vi "IFA300Command.vi"(4 "Channel Name":string, 6 "Port Name":string, 8 "ValueToSet":string, 9 "IFACommand":T2="Version", 10 "Address":i8=-1) -> (0 "String Reply":string, 1 "Error Description":string, 2 "Numeric Reply":dbl)   [LabVIEW 2021]
uses:
  IFA300CommandDescriptor.ctl
  IFA300Command.ctl
  IFA300CommandPhases.ctl
panel:
  out "CommandDescriptorOutput":T1
  out "Audit trail":string[](array[string])
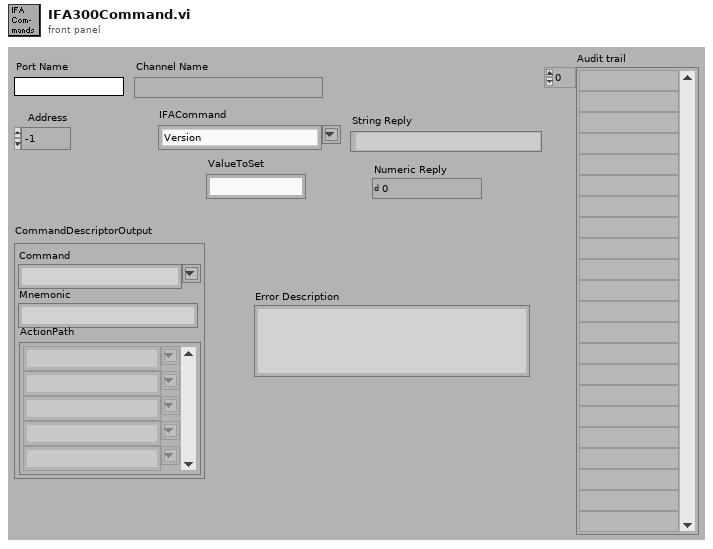
[diagram p1: front panel]
types:
  T1 = typedef "IFA300CommandDescriptor.ctl" = cluster{"Command":T2, "Mnemonic":string, "ActionPath":T3[]}
  T2 = typedef "IFA300Command.ctl" = string
  T3 = typedef "IFA300CommandPhases.ctl" = string
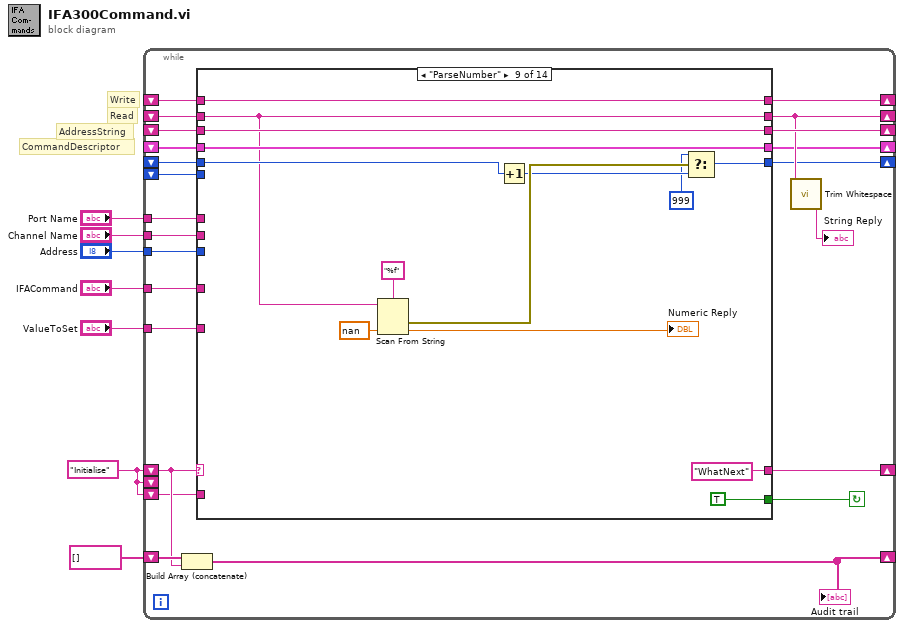
[diagram p0: block diagram]
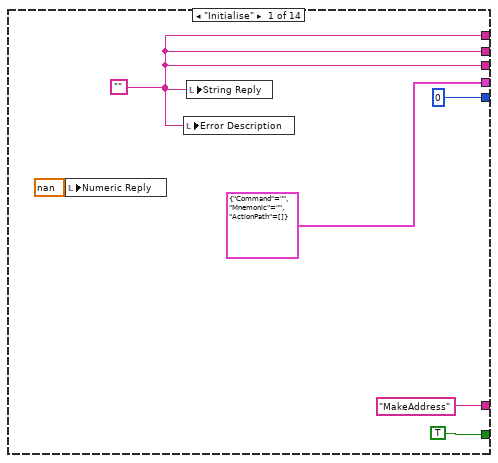
[diagram p2: hidden frame]
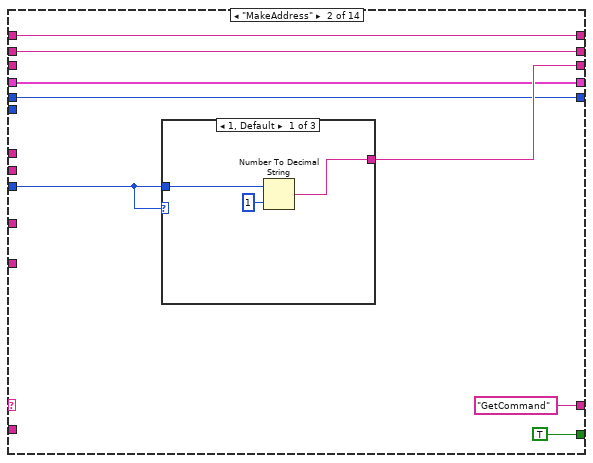
[diagram p3: hidden frame]
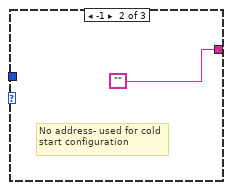
[diagram p4: hidden frame]
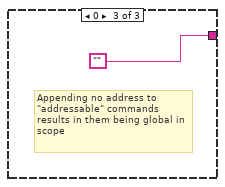
[diagram p5: hidden frame]
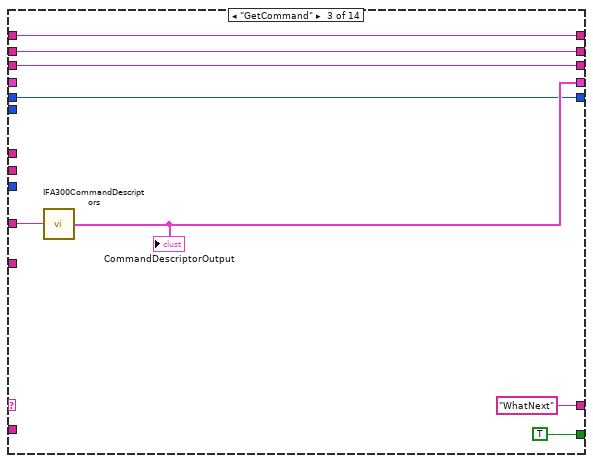
[diagram p6: hidden frame]
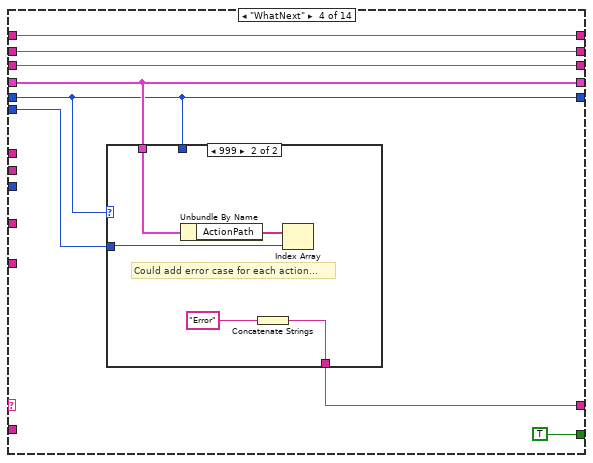
[diagram p7: hidden frame]
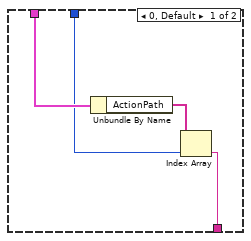
[diagram p8: hidden frame]
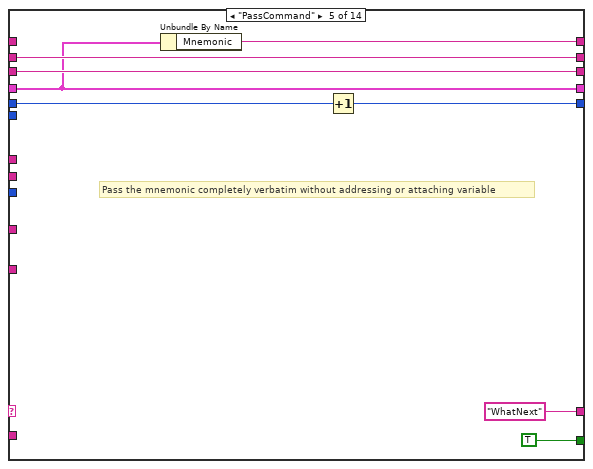
[diagram p9: hidden frame]
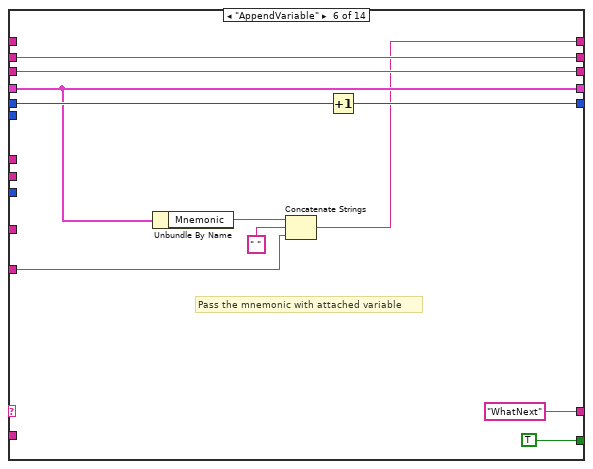
[diagram p10: hidden frame]
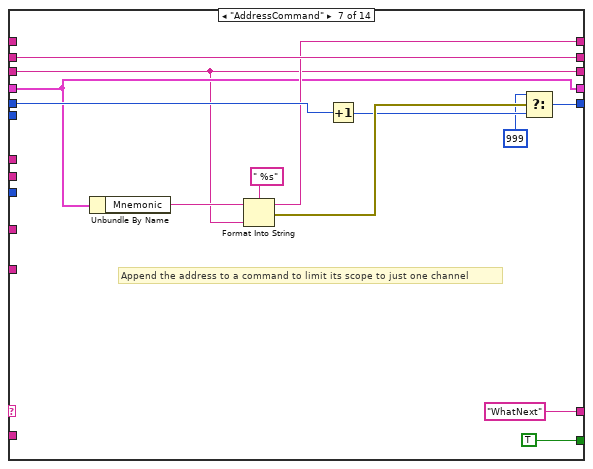
[diagram p11: hidden frame]
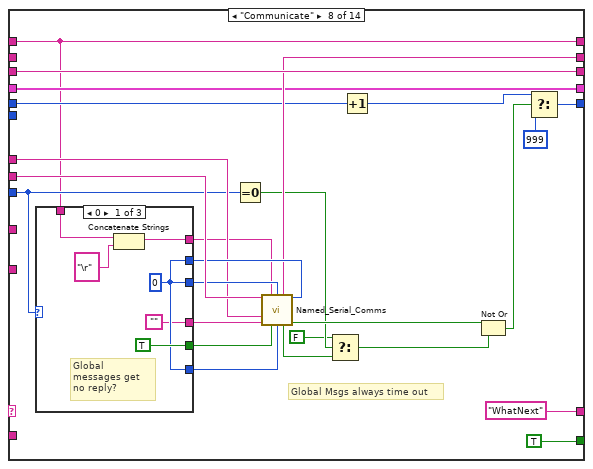
[diagram p12: hidden frame]
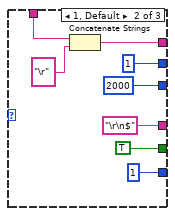
[diagram p13: hidden frame]
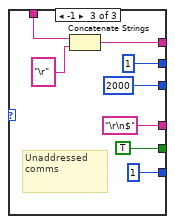
[diagram p14: hidden frame]
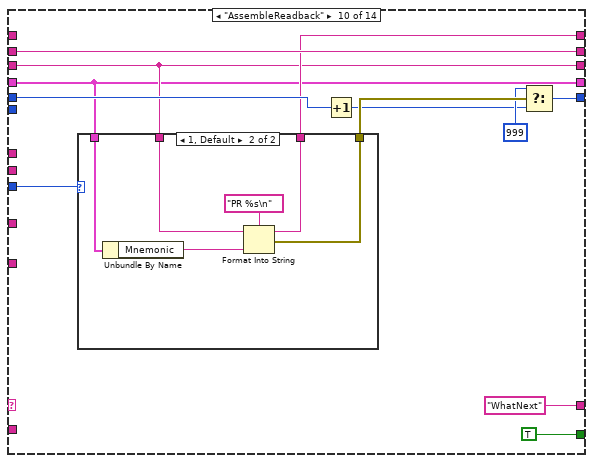
[diagram p15: hidden frame]
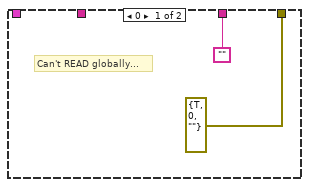
[diagram p16: hidden frame]
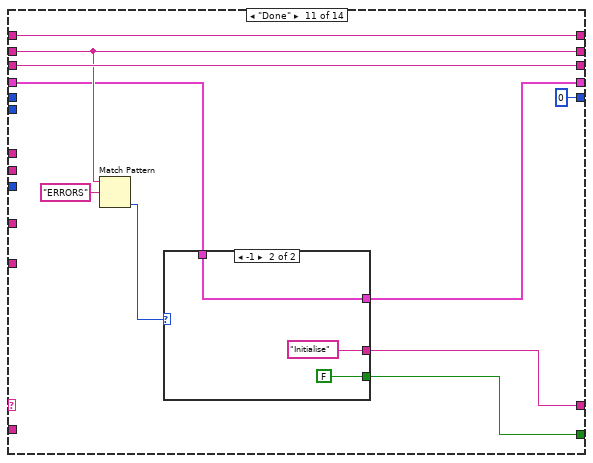
[diagram p17: hidden frame]
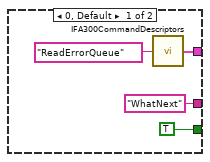
[diagram p18: hidden frame]
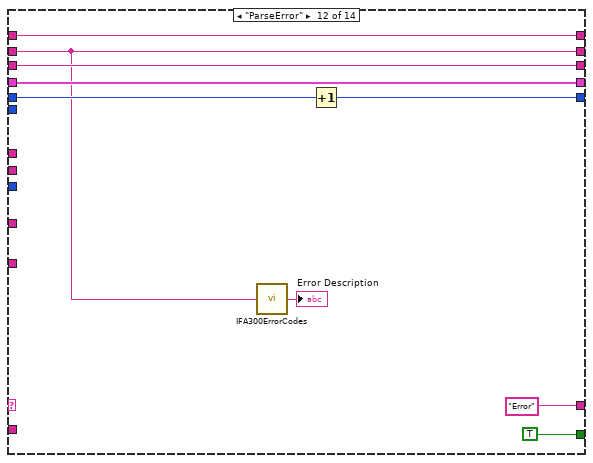
[diagram p19: hidden frame]
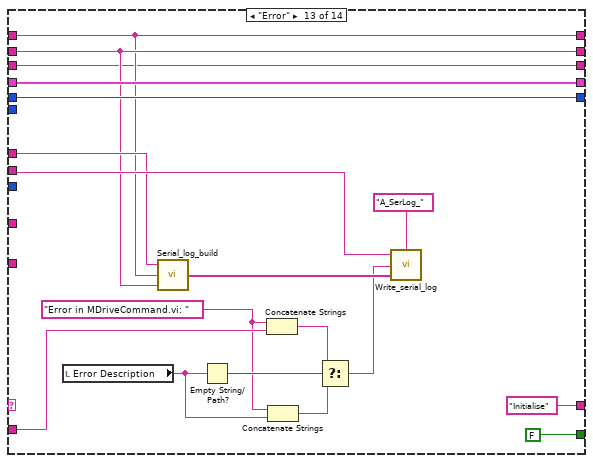
[diagram p20: hidden frame]
diagram:
  w1 = "Initialise"
  # "CommandDescriptor"
  # "AddressString"
  # "Read"
  # "Write"
  n1 = while {
    shift-right: [w18] -> _
    shift-left: w1 -> [w11]
    tunnel: "Address" -> [w30]
    tunnel: "IFACommand" -> [w29]
    tunnel: "ValueToSet" -> [w28]
    shift-right: [w27] -> _
    shift-left: _ -> [w26]
    tunnel: "Port Name" -> [w25]
    tunnel: "Channel Name" -> [w24]
    shift-right: [w16] -> _
    shift-left: _ -> [w23]
    shift-right: [w21] -> _
    shift-left: _ -> [w20]
    shift-right: [w17] -> _
    shift-left: string[] [] -> [w19]
    shift-right: [w15] -> _
    shift-left: _ -> [w14]
    shift-right: [w12] -> _
    shift-left: _ -> [w13]
    shift-left: _ -> [w10]
    shift-left: w1 -> [_]
    shift-left: w1 -> [w9]
    stop <- w22 continue-if-true
    n2 = Build Array (concatenate)(w19, w11) -> (w17:T3[])
    "Audit trail" <- w17
    n3 = case shown="\"ParseNumber\"" w11 {
      selector: w11 -> [_ _ _ _ _ _ _ _ _ _ _ _ _ w236]
      tunnel: ["MakeAddress" "GetCommand" "WhatNext" w61 "WhatNext" "WhatNext" "WhatNext" "WhatNext" "WhatNext" "WhatNext" w191 "Error" "Initialise" w236] -> w18
      tunnel: w30 -> [_ w37 _ _ _ _ _ w109 _ w171 _ _ _ _]
      tunnel: w29 -> [_ _ w54 _ _ _ _ _ _ _ _ _ _ _]
      tunnel: w28 -> [_ _ _ _ _ w83 _ _ _ _ _ _ _ _]
      tunnel: [w31 w42 w56 w64 w76 w85 w101 w108 w155 w174 w197 w208 w215 w234] -> w27
      tunnel: w26 -> [_ w42 w56 w64 _ _ _ w108 w155 _ w197 w208 w215 _]
      tunnel: w25 -> [_ _ _ _ _ _ _ w125 _ _ _ _ w224 _]
      tunnel: w24 -> [_ _ _ _ _ _ _ w131 _ _ _ _ w225 _]
      tunnel: [w31 w41 w55 w63 w82 w93 w106 w122 w161 w179 w195 w205 w216 w234] -> w16
      tunnel: w23 -> [_ w41 w55 w63 w82 w93 w106 _ w161 w179 w195 w205 w216 _]
      tunnel: [TRUE TRUE ("Continue") TRUE ("Continue") TRUE ("Continue") TRUE TRUE TRUE TRUE TRUE TRUE w192 TRUE FALSE ("Continue") FALSE] -> w22
      tunnel: [w31 w44 w53 w62 w78 w89 w94 w123 w166 w172 w196 w212 w214 w234] -> w21
      tunnel: w20 -> [_ _ w53 w62 w78 w89 w94 w123 w166 w172 w196 w212 w214 _]
      tunnel: [T1 {"Command"="", "Mnemonic"="", "ActionPath"=[]} ("CommandDescriptorOutput") w39 w51 w60 w77 w88 w99 w121 w162 w170 w189 w209 w229 w233] -> w15
      tunnel: w14 -> [_ w39 _ w60 w77 w88 w99 w121 w162 w170 w188 w209 w229 w233]
      tunnel: w13 -> [_ w38 w50 w59 w79 w90 w102 w116 w163 w175 _ w210 w228 w232]
      tunnel: [0 w38 w50 w59 w75 w87 w103 w118 w164 w176 0 ("f") w206 w228 w232] -> w12
      tunnel: w10 -> [_ _ _ w58 _ _ _ _ _ _ _ _ _ _]
      tunnel: w9 -> [_ _ _ _ _ _ _ _ _ _ _ _ w222 _]
      frame "Initialise" {
        w31 = ""
        n4 = local write "Numeric Reply"(nan ("Numeric Reply")) -> ()
        n5 = local write "Error Description"(w31) -> ()
        n6 = local write "String Reply"(w31) -> ()
      }
      frame "MakeAddress" {
        n7 = case shown="1, Default" w37 {
          tunnel: w37 -> [w46 _ _]
          tunnel: [w45 "" ""] -> w44
          frame 1, Default {
            n8 = Number To Decimal String(number=w46, width (-)=i16 1) -> (decimal integer string=w45:string)
          }
          frame -1 {
            # "No address- used for cold start configuration"
          }
          frame 0 {
            # "Appending no address to \"addressable\" commands results in them being global in scope"
          }
        }
      }
      frame "GetCommand" {
        n9 = call "IFA300CommandDescriptors.vi"("IFACommand"=w54) -> ("CommandDescriptorOutput"=w51:T1)  [unwired: 4 out]
        "CommandDescriptorOutput" <- w51
      }
      frame "WhatNext" {
        n10 = case shown="999" w59 {
          tunnel: [w68 w71] -> w61
          tunnel: w60 -> [w67 w72]
          tunnel: w59 -> [w66 _]
          tunnel: w58 -> [_ w73]
          frame 0, Default {
            n11 = Unbundle By Name(w67) -> ("ActionPath"=w69:T3[])
            n12 = Index Array(array=w69, index=w66) -> (element=w68:T3)
          }
          frame 999 {
            # "Could add error case for each action..."
            n13 = Unbundle By Name(w72) -> ("ActionPath"=w74:T3[])
            n14 = Concatenate Strings("Error") -> (w71:string)
            n15 = Index Array(array=w74, index=w73) -> ()  [unwired: 1 out]
          }
        }
      }
      frame "PassCommand" {
        # "Pass the mnemonic completely verbatim without addressing or attaching variable"
        n16 = Unbundle By Name(w77) -> ("Mnemonic"=w76:string)
        n17 = Increment(x=w79) -> (x+1=w75:i32)
      }
      frame "AppendVariable" {
        # "Pass the mnemonic with attached variable"
        n18 = Unbundle By Name(w88) -> ("Mnemonic"=w86:string)
        n19 = Concatenate Strings(w86, " " ("string"), w83) -> (w85:string)
        n20 = Increment(x=w90) -> (x+1=w87:i32)
      }
      frame "AddressCommand" {
        # "Append the address to a command to limit its scope to just one channel"
        n21 = Unbundle By Name(w99) -> ("Mnemonic"=w95:string)
        n22 = Format Into String(format string=" %s", initial string=w95, w94) -> (resulting string=w101:string, error out=w98:errorcluster)  [unwired: 1 in]
        n23 = Increment(x=w102) -> (x+1=w97:i32)
        n24 = Select(t=999 ("f"), s=w98, f=w97) -> (s? t:f=w103:i32)
      }
      frame "Communicate" {
        # "Global Msgs always time out"
        n25 = case shown="0" w109 {
          tunnel: ["" "\r\n$" "\r\n$"] -> w130
          tunnel: [w136 1 ("Terminate Count") 1 ("Terminate Count")] -> w129
          tunnel: [w136 u32 2000 ("Timeout/ms") u32 2000 ("Timeout/ms")] -> w128
          tunnel: [TRUE ("Log Errors?") TRUE ("Log Errors?") TRUE ("Log Errors?")] -> w127
          tunnel: [w136 1 ("!Error retries") 1 ("!Error retries")] -> w126
          tunnel: w108 -> [w132 w140 w148]
          tunnel: [w133 w139 w147] -> w107
          frame 0 {
            w136 = 0 ("!Error retries")
            # "Global messages get no reply?"
            n26 = Concatenate Strings(w132, "\r" ("string")) -> (w133:string)
          }
          frame 1, Default {
            n27 = Concatenate Strings(w140, "\r" ("string")) -> (w139:string)
          }
          frame -1 {
            # "Unaddressed comms"
            n28 = Concatenate Strings(w148, "\r" ("string")) -> (w147:string)
          }
        }
        n29 = Equal To 0?(x=w109) -> (x = 0?=w112:bool)
        n30 = call "Named_Serial_Comms.vi"("Channel Name"=w131, "Write"=w107, "Timeout/ms"=w128, "!Error retries"=w126, "Port Name"=w125, "Term Grep"=w130, "Log Errors?"=w127, "Terminate Count"=w129) -> ("Read"=w122:string, "Timed out"=w111:bool, "Serial Error"=w119:bool)  [unwired: 1 in, 4 out]
        n31 = Select(t=FALSE, s=w112, f=w111) -> (s? t:f=w113:bool)
        n32 = Increment(x=w116) -> (x+1=w115:i32)
        n33 = Not Or(1:w113, 2:w119) -> (0:w117:bool)
        n34 = Select(t=w115, s=w117, f=999) -> (s? t:f=w118:i32)
      }
      frame "ParseNumber" {
        n35 = Scan From String(format string="%f", input string=w161, default 1=nan ("default value 1")) -> (error out=w159:errorcluster, output 1=→"Numeric Reply":dbl)  [unwired: 2 in, 2 out]
        n36 = Increment(x=w163) -> (x+1=w158:i32)
        n37 = Select(t=999, s=w159, f=w158) -> (s? t:f=w164:i32)
      }
      frame "AssembleReadback" {
        n38 = case shown="1, Default" w171 {
          tunnel: w170 -> [_ w187]
          tunnel: ["" w186] -> w174
          tunnel: [errorcluster {"status"=TRUE, "code"=0, "source"=""} ("error IO") w185] -> w173
          tunnel: w172 -> [_ w184]
          frame 0 {
            # "Can't READ globally..."
          }
          frame 1, Default {
            n39 = Unbundle By Name(w187) -> ("Mnemonic"=w183:string)
            n40 = Format Into String(format string="PR %s\n", initial string=w184, w183) -> (resulting string=w186:string, error out=w185:errorcluster)  [unwired: 1 in]
          }
        }
        n41 = Increment(x=w175) -> (x+1=w168:i32)
        n42 = Select(t=999 ("f"), s=w173, f=w168) -> (s? t:f=w176:i32)
      }
      frame "Done" {
        n43 = Match Pattern(string=w195, regular expression="ERRORS") -> (offset past match=w190:i32)  [unwired: 4 out]
        n44 = case shown="-1" w190 {
          tunnel: [TRUE ("Continue") FALSE ("Continue")] -> w192
          tunnel: ["WhatNext" "Initialise"] -> w191
          tunnel: [w200 w202] -> w189
          tunnel: w188 -> [_ w202]
          frame 0, Default {
            n45 = call "IFA300CommandDescriptors.vi"("IFACommand"=T2 "ReadErrorQueue" ("MDriveCommand")) -> ("CommandDescriptorOutput"=w200:T1)  [unwired: 4 out]
          }
          frame -1 {
          }
        }
      }
      frame "ParseError" {
        n46 = call "IFA300ErrorCodes.vi"("Error Code"=w205) -> ("Error Description"=→"Error Description":string)  [unwired: 4 out]
        n47 = Increment(x=w210) -> (x+1=w206:i32)
      }
      frame "Error" {
        w219 = "Error in MDriveCommand.vi: " ("string")
        n48 = local read "Error Description"() -> (w218:string)
        n49 = call "Serial_log_build.vi"("Read"=w216, "Write String"=w215, "Port Name"=w224) -> ("Output Array"=w226:string[])
        n50 = Empty String/Path?(string/path=w218) -> (empty?=w223:bool)
        n51 = Concatenate Strings(w219, w222) -> (w221:string)
        n52 = Concatenate Strings(w219, w218) -> (w220:string)
        n53 = Select(t=w221, s=w223, f=w220) -> (s? t:f=w217:string)
        n54 = call "Write_serial_log.vi"("Log Type"="A_SerLog_", "Log Array"=w226, "Header message"=w217, "Channel Name"=w225) -> ()  [unwired: 1 out]
      }
      frame "NoMatch", Default {
        w234 = ""
        n55 = One Button Dialog(message="Case not found in MDriveCommands.vi", button name ("OK")="Oh Bugger...") -> ()  [unwired: 1 out]
      }
    }
    n56 = call <vilib>:"Trim Whitespace.vi"("string"=w16) -> ("trimmed string"=→"String Reply":string)  [unwired: 1 in]
  }
